vi "operacion_con_enum.vi"() -> ()   [LabVIEW 2020]
panel:
  in  "Enum":T1(ring)
  out "Resultados":dbl
  in  "Valor 2":dbl
  in  "Valor 1":dbl
  in  "Suma":bool
  out "Resultado":dbl
  in  "Valor 2":dbl
  in  "Valor 1":dbl
  # "Resta"
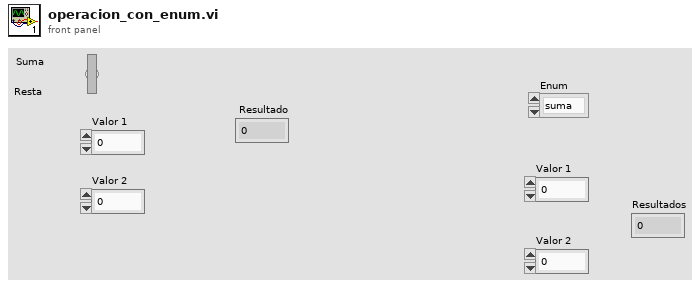
[diagram p1: front panel]
types:
  T1 = enum16{"suma", "resta", "multiplicacion", "division"}
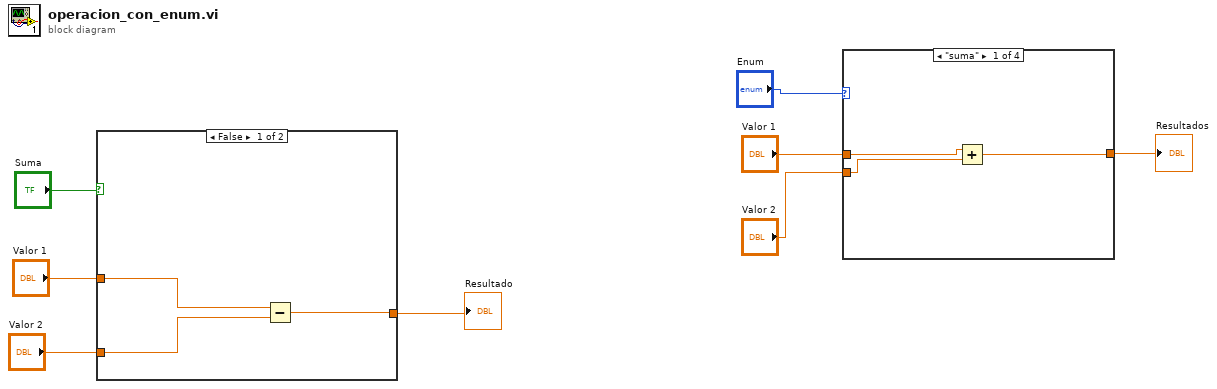
[diagram p0: block diagram]
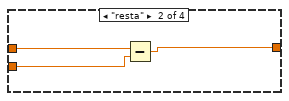
[diagram p2: hidden frame]
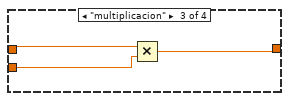
[diagram p3: hidden frame]
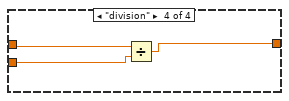
[diagram p4: hidden frame]
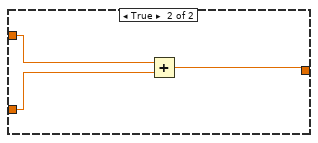
[diagram p5: hidden frame]
diagram:
  n1 = case shown="False" "Suma" {
    tunnel: "Valor 1" -> [w11 w13]
    tunnel: "Valor 2" -> [w10 w12]
    tunnel: [w9 w14] -> w6
    frame False {
      n2 = Subtract(x=w11, y=w10) -> (x-y=w9:dbl)
    }
    frame True {
      n3 = Add(x=w13, y=w12) -> (x+y=w14:dbl)
    }
  }
  "Resultado" <- w6
  n4 = case shown="\"suma\"" "Enum" {
    tunnel: "Valor 1" -> [w17 w20 w23 w26]
    tunnel: "Valor 2" -> [w16 w19 w22 w25]
    tunnel: [w15 w18 w21 w24] -> w2
    frame "suma" {
      n5 = Add(x=w17, y=w16) -> (x+y=w15:dbl)
    }
    frame "resta" {
      n6 = Subtract(x=w20, y=w19) -> (x-y=w18:dbl)
    }
    frame "multiplicacion" {
      n7 = Multiply(x=w23, y=w22) -> (x*y=w21:dbl)
    }
    frame "division" {
      n8 = Divide(x=w26, y=w25) -> (x/y=w24:dbl)
    }
  }
  "Resultados" <- w2
